vi "Load COM Info.vi"(11 "Serial Instrument":T1) -> (3 "COM Port":refnum<visa-resource-name>)   [LabVIEW 2015, in "RDS Configuration Library.lvlib"]
uses:
  Configuration Library/RDS Configuration Library.lvlib
  RDS Instrument Enums.ctl
  COM Port Table.ctl
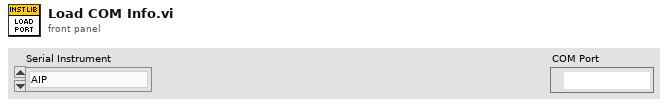
[diagram p1: front panel]
types:
  T1 = typedef "RDS Configuration Library.lvlib/RDS Instrument Enums.ctl" = enum16{"AIP", "GPS", "Compass", "PORT Motor", "STBD Motor", "LSR", "Depth Transducer", "BTB"}
  T2 = typedef "RDS Configuration Library.lvlib/COM Port Table.ctl" = cluster{"LSR":refnum<visa-resource-name>, "MCB Port":refnum<visa-resource-name>, "MCB STBD":refnum<visa-resource-name>, "Depth Transducer":refnum<visa-resource-name>, "Compass":refnum<visa-resource-name>, "GPS":refnum<visa-resource-name>, "Battery":refnum<visa-resource-name>, "AIP":refnum<visa-resource-name>}
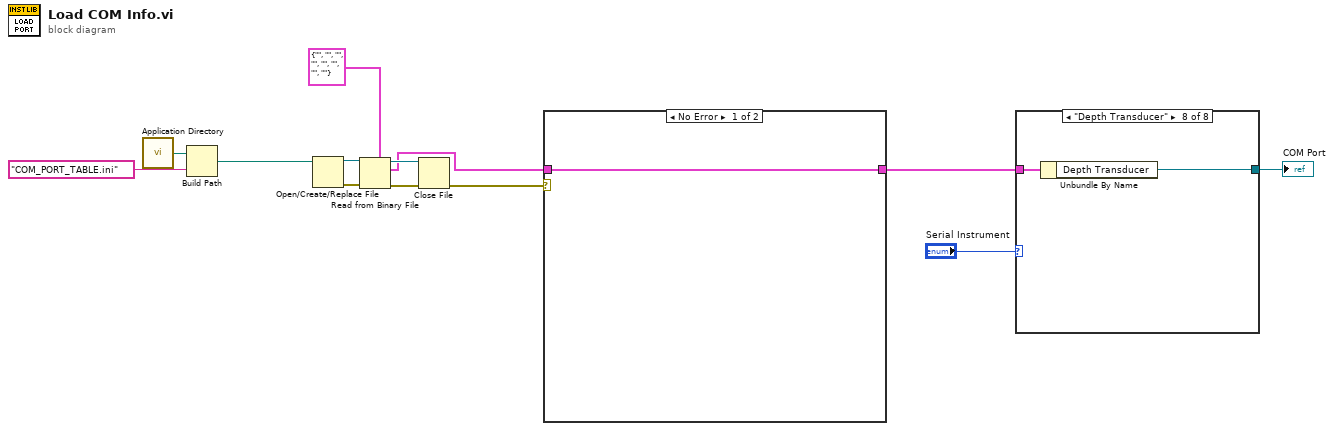
[diagram p0: block diagram]
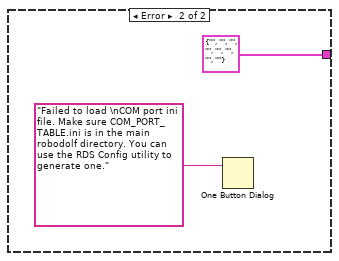
[diagram p2: hidden frame]
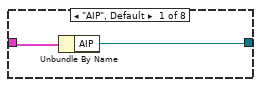
[diagram p3: hidden frame]
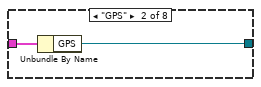
[diagram p4: hidden frame]
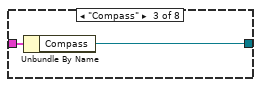
[diagram p5: hidden frame]
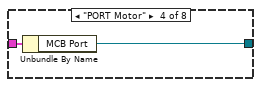
[diagram p6: hidden frame]
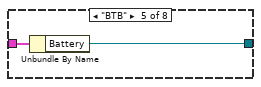
[diagram p7: hidden frame]
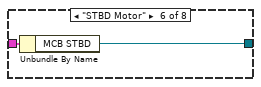
[diagram p8: hidden frame]
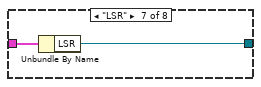
[diagram p9: hidden frame]
diagram:
  n1 = call <vilib>:"Application Directory.vi"() -> ("Application Directory"=w13:path)
  n2 = Build Path(base path=w13, name or relative path="COM_PORT_TABLE.ini") -> (appended path=w3:path)
  n3 = Open/Create/Replace File(file path (use dialog)=w3) -> (refnum out=w5:refnum<file>, error out=w6:errorcluster)  [unwired: 5 in, 1 out]
  n4 = Read from Binary File(5:T2 {"LSR"="", "MCB Port"="", "MCB STBD"="", "Depth Transducer"="", "Compass"="", "GPS"="", "Battery"="", "AIP"=""} ("COM Port Table"), 8:w6, 11:w5) -> (0:w7:errorcluster, 2:w1:T2, 3:w8:refnum<file>)  [unwired: 3 in, 1 out]
  n5 = Close File(refnum=w8, error in=w7) -> (error out=w4:errorcluster)  [unwired: 1 out]
  n6 = case shown="No Error" w4 {
    tunnel: [w14 T2 {"LSR"="", "MCB Port"="", "MCB STBD"="", "Depth Transducer"="", "Compass"="", "GPS"="", "Battery"="", "AIP"=""} ("COM Port Table")] -> w9
    tunnel: w1 -> [w14 _]
    frame No Error {
    }
    frame Error {
      n7 = One Button Dialog(message="Failed to load \nCOM port ini file. Make sure COM_PORT_TABLE.ini is in the main robodolf directory. You can use the RDS Config utility to generate one.") -> ()  [unwired: 1 in, 1 out]
    }
  }
  n8 = case shown="\"Depth Transducer\"" "Serial Instrument" {
    tunnel: w9 -> [w18 w20 w22 w24 w26 w28 w30 w32]
    tunnel: [w17 w19 w21 w23 w25 w27 w29 w31] -> w10
    frame "AIP", Default {
      n9 = Unbundle By Name(w18) -> ("AIP"=w17:refnum<visa-resource-name>)
    }
    frame "GPS" {
      n10 = Unbundle By Name(w20) -> ("GPS"=w19:refnum<visa-resource-name>)
    }
    frame "Compass" {
      n11 = Unbundle By Name(w22) -> ("Compass"=w21:refnum<visa-resource-name>)
    }
    frame "PORT Motor" {
      n12 = Unbundle By Name(w24) -> ("MCB Port"=w23:refnum<visa-resource-name>)
    }
    frame "BTB" {
      n13 = Unbundle By Name(w26) -> ("Battery"=w25:refnum<visa-resource-name>)
    }
    frame "STBD Motor" {
      n14 = Unbundle By Name(w28) -> ("MCB STBD"=w27:refnum<visa-resource-name>)
    }
    frame "LSR" {
      n15 = Unbundle By Name(w30) -> ("LSR"=w29:refnum<visa-resource-name>)
    }
    frame "Depth Transducer" {
      n16 = Unbundle By Name(w32) -> ("Depth Transducer"=w31:refnum<visa-resource-name>)
    }
  }
  "COM Port" <- w10
